vi "ke2000 Read Single Example.vi"() -> ()   [LabVIEW 2010]
doc: "This example shows how to select a function, use a bus trigger, and read a measurement."
uses:
  <instrlib>/ke2000/ke2000.llb/ke2000 Configure Measurement.vi
panel:
  out "Units":string
  out "Measurement":dbl
  in  "Measure":bool
  in  "Function (0: DC Volts)":u16(ring) items=["DC Volts", "AC Volts", "DC Current", "AC Current", "2-Wire Resistance", "4-Wire Resistance"]
  in  "VISA resource name":refnum<visa-resource-name>="GPIB::16"
  # "This example shows how to select a function, \nuse a bus trigger, and read a measurement.\n\nInstructions:\n1. Select a function.\n2. Run the VI\n3. Press the \"Measure\" button to take a measurement."
  # "© 2003, National Instruments, Corporation.  All Rights Reserved."
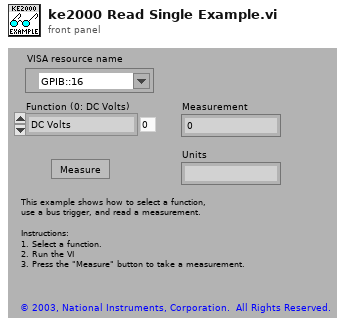
[diagram p1: front panel]
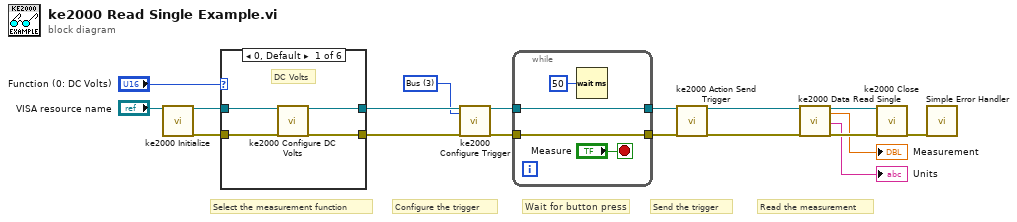
[diagram p0: block diagram]
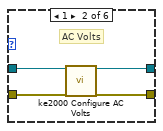
[diagram p2: hidden frame]
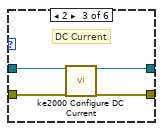
[diagram p3: hidden frame]
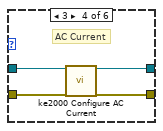
[diagram p4: hidden frame]
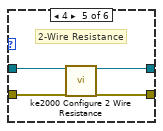
[diagram p5: hidden frame]
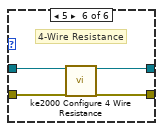
[diagram p6: hidden frame]
diagram:
  w7 = u16 3 items=["Immediate", "Timer", "Manual", "Bus", "External"] ("Source (0: Immediate)")
  # "Read the measurement"
  # "Send the trigger"
  # "Wait for button press"
  # "Configure the trigger"
  # "Select the measurement function"
  n1 = call <instrlib>:"ke2000 Initialize.vi"("VISA resource name"="VISA resource name") -> ("VISA resource name out"=w15:refnum<visa-resource-name>, "error out"=w18:errorcluster)  [unwired: 17 in]
  n2 = case shown="0, Default" "Function (0: DC Volts)" {
    tunnel: w18 -> [w22 w26 w30 w34 w38 w42]
    tunnel: w15 -> [w21 w25 w29 w33 w37 w41]
    tunnel: [w20 w24 w28 w32 w36 w40] -> w12
    tunnel: [w19 w23 w27 w31 w35 w39] -> w11
    frame 0, Default {
      # "DC Volts"
      n3 = call-poly <instrlib>:"ke2000 Configure DC Volts.vi"("VISA resource name"=w21, "error in (no error)"=w22) -> ("VISA resource name out"=w19:refnum<visa-resource-name>, "error out"=w20:errorcluster)  [unwired: 16 in]
    }
    frame 1 {
      # "AC Volts"
      n4 = call-poly <instrlib>:"ke2000 Configure AC Volts.vi"("VISA resource name"=w25, "error in (no error)"=w26) -> ("VISA resource name out"=w23:refnum<visa-resource-name>, "error out"=w24:errorcluster)  [unwired: 16 in]
    }
    frame 2 {
      # "DC Current"
      n5 = call-poly <instrlib>:"ke2000 Configure DC Current.vi"("VISA resource name"=w29, "error in (no error)"=w30) -> ("VISA resource name out"=w27:refnum<visa-resource-name>, "error out"=w28:errorcluster)  [unwired: 16 in]
    }
    frame 3 {
      # "AC Current"
      n6 = call-poly <instrlib>:"ke2000 Configure AC Current.vi"("VISA resource name"=w33, "error in (no error)"=w34) -> ("VISA resource name out"=w31:refnum<visa-resource-name>, "error out"=w32:errorcluster)  [unwired: 16 in]
    }
    frame 4 {
      # "2-Wire Resistance"
      n7 = call-poly <instrlib>:"ke2000 Configure 2 Wire Resistance.vi"("VISA resource name"=w37, "error in (no error)"=w38) -> ("VISA resource name out"=w35:refnum<visa-resource-name>, "error out"=w36:errorcluster)  [unwired: 16 in]
    }
    frame 5 {
      # "4-Wire Resistance"
      n8 = call-poly <instrlib>:"ke2000 Configure 4 Wire Resistance.vi"("VISA resource name"=w41, "error in (no error)"=w42) -> ("VISA resource name out"=w39:refnum<visa-resource-name>, "error out"=w40:errorcluster)  [unwired: 16 in]
    }
  }
  n9 = call <instrlib>:"ke2000 Configure Trigger.vi"("VISA resource name"=w11, "Source (0: Immediate)"=w7, "error in (no error)"=w12) -> ("VISA resource name out"=w6:refnum<visa-resource-name>, "error out"=w5:errorcluster)  [unwired: 15 in]
  n10 = while {
    tunnel: w6 -> [w46]
    tunnel: w5 -> [w45]
    tunnel: [w46] -> w4
    tunnel: [w45] -> w3
    stop <- "Measure" stop-if-true
    n11 = Wait (ms)(milliseconds to wait=u32 50) -> ()  [unwired: 1 out]
  }
  n12 = call <instrlib>:"ke2000 Action Send Trigger.vi"("VISA resource name"=w4, "error in (no error)"=w3) -> ("VISA resource name out"=w1:refnum<visa-resource-name>, "error out"=w2:errorcluster)  [unwired: 16 in]
  n13 = call <instrlib>:"ke2000 Data Read Single.vi"("VISA resource name"=w1, "error in (no error)"=w2) -> ("VISA resource name out"=w16:refnum<visa-resource-name>, "Measurement"=→"Measurement":dbl, "Units"=→"Units":string, "error out"=w17:errorcluster)  [unwired: 13 in, 1 out]
  n14 = call <instrlib>:"ke2000 Close.vi"("VISA resource name"=w16, "error in (no error)"=w17) -> ("error out"=w14:errorcluster)  [unwired: 17 in]
  n15 = call <vilib>:"Simple Error Handler.vi"("error in (no error)"=w14) -> ()  [unwired: 4 in, 5 out]
